vi "Two Processes.vi"() -> ()   [LabVIEW 2010]
doc: "This VI demonstrates two processes running in parallel."
panel:
  in  "stop 2":bool
  out "Input Data":dbl(graph)
  in  "stop":bool
  out "Value > 0?":bool
  out "Current Time":timestamp format="%<%I:%M:%S %p\n%x>T"
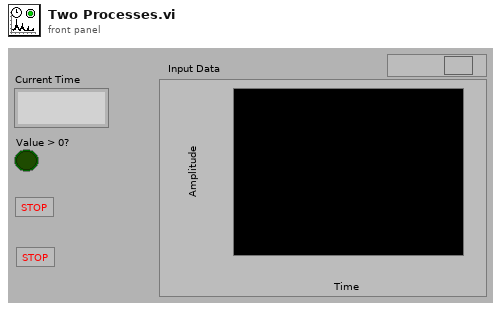
[diagram p1: front panel]
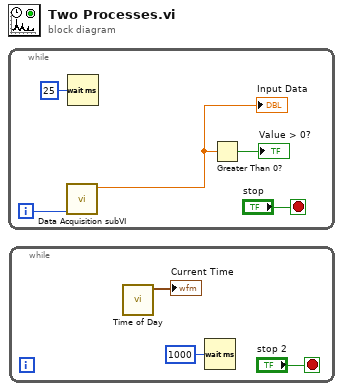
[diagram p0: block diagram]
diagram:
  n1 = while {
    i -> [w2]
    stop <- "stop" stop-if-true
    n2 = call "Data Acquisition subVI.vi"("Numeric in"=w2) -> ("Numeric out"=w4:dbl)  [unwired: 10 in]
    "Input Data" <- w4
    n3 = Wait (ms)(milliseconds to wait=u32 25) -> ()  [unwired: 1 out]
    n4 = Greater Than 0?(x=w4) -> (x > 0?=→"Value > 0?":bool)
  }
  n5 = while {
    stop <- "stop 2" stop-if-true
    n6 = call "Time of Day.vi"() -> ("current time"=→"Current Time":timestamp)  [unwired: 11 in]
    n7 = Wait (ms)(milliseconds to wait=u32 1000) -> ()  [unwired: 1 out]
  }
